vi "Set Fixed-Point Raw Data.vi"(8 "Error In":errorcluster) -> (0 "error out":errorcluster, 1 "Value Calculation + Write Graph":dbl[](graph), 2 "Write Average":dbl, 3 "Value Calculation + Write Average":dbl)   [LabVIEW 2018]
uses:
  NiFpga.dll
panel:
  out "Write Graph":dbl[](graph)
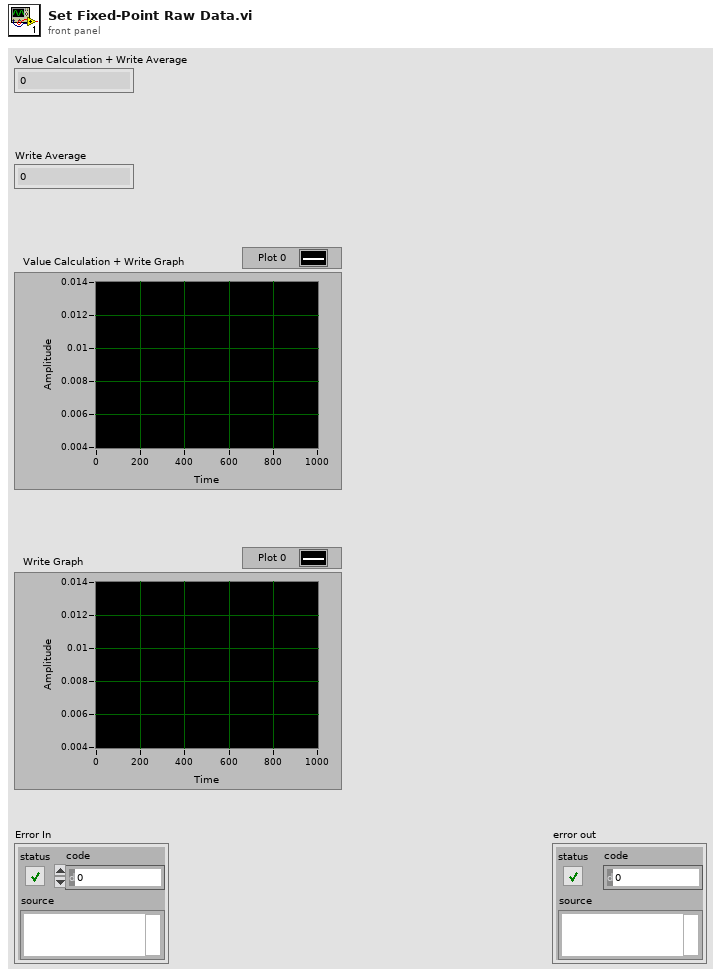
[diagram p1: front panel]
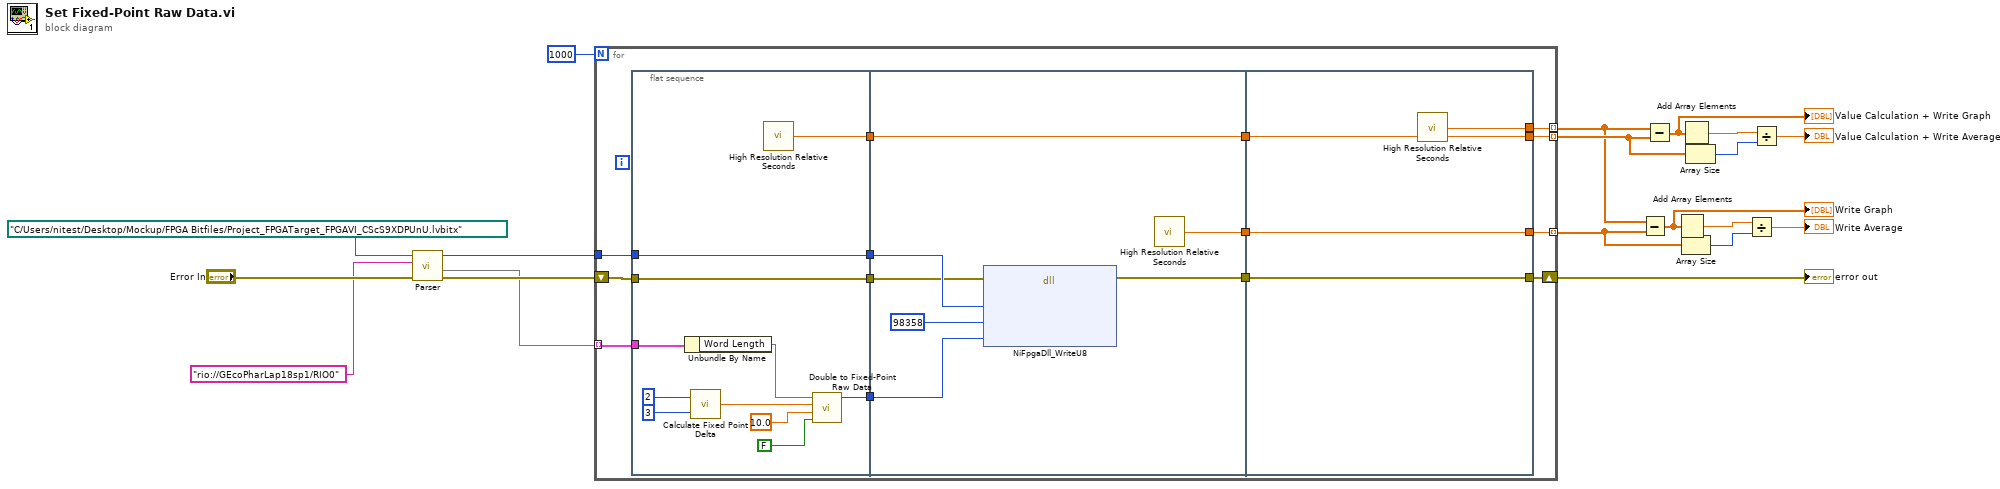
[diagram p0: block diagram]
diagram:
  n1 = call "Parser.vi"("error in (no error)"="Error In", "RIO device address"="rio://GEcoPharLap18sp1/RIO0" ("Device address"), "bitfile path"=path "C:/Users/nitest/Desktop/Mockup/FPGA Bitfiles/Project_FPGATarget_FPGAVI_CScS9XDPUnU.lvbitx" ("Bitfile path")) -> ("error out"=w16:errorcluster, 1:w1, "session out"=w14:u64)  [unwired: 5 in, 1 out]
  n2 = for {
    N: 1000 -> [_]
    tunnel: w14 -> [w32]
    shift-right: [w23] -> w19
    shift-left: w16 -> [w33]
    tunnel: [w26] -> w8 mode=indexing
    tunnel: [w25] -> w2 mode=indexing
    tunnel: [w21] -> w3 mode=indexing
    tunnel: w1 -> [w20] mode=indexing
    n3 = flat-sequence {
      tunnel: w32 -> [w43]
      tunnel: w33 -> [w44]
      tunnel: [w44] -> w31
      tunnel: [w43] -> w30
      tunnel: [w42] -> w28
      tunnel: [w39] -> w27
      tunnel: w20 -> [w38]
      tunnel: w31 -> [w48]
      tunnel: w30 -> [w50]
      tunnel: [w51] -> w29
      tunnel: w28 -> [w51]
      tunnel: w27 -> [w47]
      tunnel: [w46] -> w24
      tunnel: [w45] -> w22
      tunnel: w29 -> [w55]
      tunnel: [w55] -> w26
      tunnel: [w54] -> w25
      tunnel: w24 -> [w53]
      tunnel: [w53] -> w23
      tunnel: w22 -> [w52]
      tunnel: [w52] -> w21
      frame #0 {
        n4 = Unbundle By Name(w38) -> ("Word Length"=w37)
        n5 = call "Calculate Fixed Point Delta.vi"("WordLength"=i8 3, "IntegerWordLength"=i8 2) -> ("delta"=w36:dbl)
        n6 = call <vilib>:"High Resolution Relative Seconds.vi"() -> ("relative seconds"=w42:dbl)
        n7 = call "Double to Fixed-Point Raw Data.vi"("isSigned?"=FALSE, "data"=10.0, "delta"=w36, "word length"=w37) -> ("Value"=w39:i64)  [unwired: 7 in]
      }
      frame #1 {
        n8 = dll-call lib="NiFpga.*" fn="NiFpgaDll_WriteU8"(error in=w48, "session"=w50, "control"=u32 98358, "value"=w47) -> (error out=w46:errorcluster)  [unwired: 6 in, 1 out]
        n9 = call <vilib>:"High Resolution Relative Seconds.vi"() -> ("relative seconds"=w45:dbl)
      }
      frame #2 {
        n10 = call <vilib>:"High Resolution Relative Seconds.vi"() -> ("relative seconds"=w54:dbl)
      }
    }
  }
  "error out" <- w19
  n11 = Subtract(x=w2, y=w3) -> (x-y=w7:dbl[])
  "Write Graph" <- w7
  n12 = Subtract(x=w2, y=w8) -> (x-y=w9:dbl[])
  "Value Calculation + Write Graph" <- w9
  n13 = Add Array Elements(numeric array=w7) -> (sum=w4:dbl)
  n14 = Array Size(array=w3) -> (size(s)=w5:i32)
  n15 = Add Array Elements(numeric array=w9) -> (sum=w12:dbl)
  n16 = Array Size(array=w8) -> (size(s)=w11:i32)
  n17 = Divide(x=w4, y=w5) -> (x/y=→"Write Average":dbl)
  n18 = Divide(x=w12, y=w11) -> (x/y=→"Value Calculation + Write Average":dbl)
